vi "Create or Update DB.vi"(8 "error in (no error)":errorcluster, 10 "Nombre":string, 11 "Contabilidad in":refnum<class "Contabilidad.lvclass">) -> (0 "error out":errorcluster, 3 "Contabilidad out":refnum<class "Contabilidad.lvclass">)   [LabVIEW 2021, in "Contabilidad.lvlib" / "Contabilidad.lvclass"]
uses:
  Contabilidad.lvclass
  <vilib>/drjdpowell/SQLite Library/SQL Connection/Open (path).vi
  <vilib>/drjdpowell/SQLite Library/SQL Connection/Open (string).vi
  <vilib>/AdvancedString/Path To Command Line String.vi
  <vilib>/drjdpowell/SQLite Library/SQL Connection/Execute SQL (No results).vi
  <vilib>/drjdpowell/SQLite Library/SQL Connection/Connection.lvclass
  Contabilidad.lvclass/Contabilidad.ctl
  <vilib>/drjdpowell/SQLite Library/SQLite.lvlib
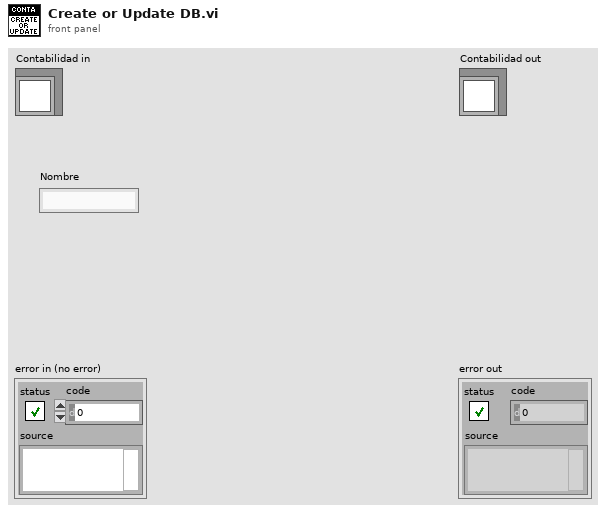
[diagram p1: front panel]
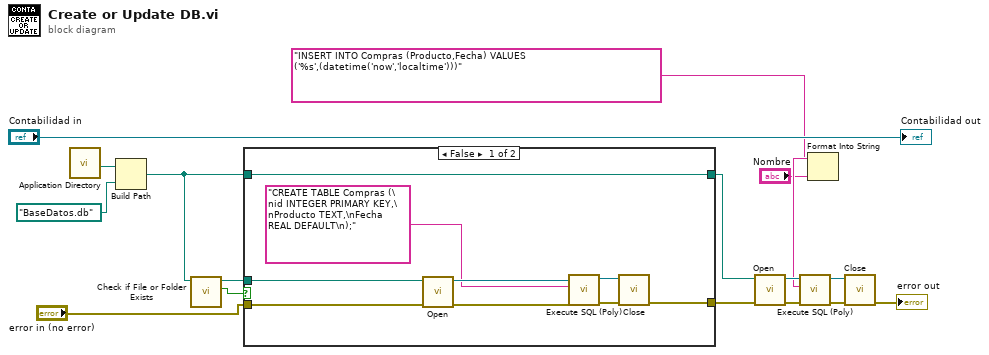
[diagram p0: block diagram]
diagram:
  n1 = call <vilib>:"Application Directory.vi"() -> ("Application Directory"=w16:path)
  n2 = Build Path(base path=w16, name or relative path=path "BaseDatos.db") -> (appended path=w4:path)
  n3 = call <vilib>:"Check if File or Folder Exists.vi"("path"=w4) -> ("file or folder exists?"=w13:bool, "dup path"=w14:path)  [unwired: 8 in, 1 out]
  n4 = case shown="False" w13 {
    tunnel: w14 -> [w26 _]
    tunnel: "error in (no error)" -> [w21 w28]
    tunnel: [w20 w28] -> w2
    tunnel: w4 -> [w18 w27]
    tunnel: [w18 w27] -> w3
    frame False {
      n5 = call-poly <vilib>:"Open.vi"("error in (no error)"=w21, "db file"=w26) -> ("error out"=w25:errorcluster, "SQLite Connection"=w24:refnum<class "Connection.lvclass">)  [unwired: 8 in]
      n6 = call-poly <vilib>:"Execute SQL (Poly).vi"("error in (no error)"=w25, "SQL"="CREATE TABLE Compras (\nid INTEGER PRIMARY KEY,\nProducto TEXT,\nFecha REAL DEFAULT\n);", "SQLite Connection in"=w24) -> ("error out"=w23:errorcluster, "SQLite Connection"=w22:refnum<class "Connection.lvclass">)  [unwired: 7 in]
      n7 = call-dynamic "Close.vi"("error in (no error)"=w23, "SQLite Connection in"=w22) -> ("error out"=w20:errorcluster)  [unwired: 9 in]
    }
    frame True {
    }
  }
  n8 = call-poly <vilib>:"Open.vi"("error in (no error)"=w2, "db file"=w3) -> ("error out"=w11:errorcluster, "SQLite Connection"=w10:refnum<class "Connection.lvclass">)  [unwired: 8 in]
  n9 = Format Into String(format string="INSERT INTO Compras (Producto,Fecha) VALUES ('%s',(datetime('now','localtime')))", "Nombre") -> (resulting string=w7:string)  [unwired: 2 in, 1 out]
  n10 = call-poly <vilib>:"Execute SQL (Poly).vi"("error in (no error)"=w11, "SQL"=w7, "SQLite Connection in"=w10) -> ("error out"=w9:errorcluster, "SQLite Connection"=w8:refnum<class "Connection.lvclass">)  [unwired: 7 in]
  n11 = call-dynamic "Close.vi"("error in (no error)"=w9, "SQLite Connection in"=w8) -> ("error out"=→"error out":errorcluster)  [unwired: 9 in]
  "Contabilidad out" <- "Contabilidad in"
